vi "Add Server Information Refnums.vi"(8 "error in (no error)":errorcluster, 9 "Server Information Controls":refnum<vi>[](array[refnum]), 10 "Server URL":refnum<k21>, 11 "Map In":variant) -> (0 "error out":errorcluster, 3 "Map Out":variant)   [LabVIEW 2024]
doc: "Adds the mapping relationship between the server information variable URL and the control refnum to the map."
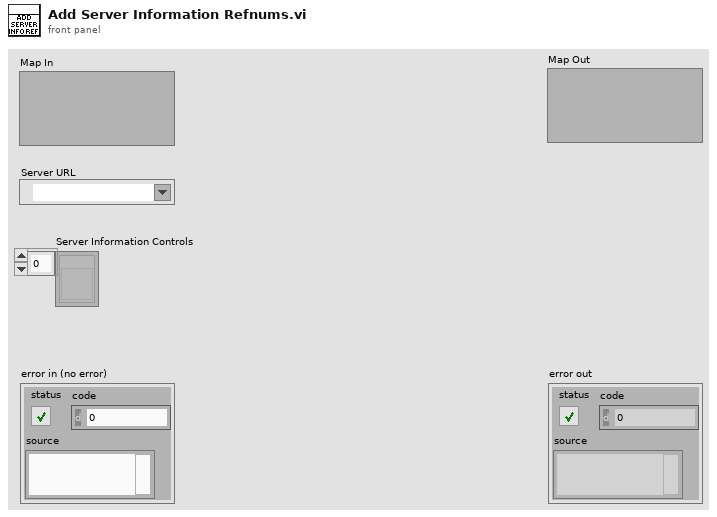
[diagram p1: front panel]
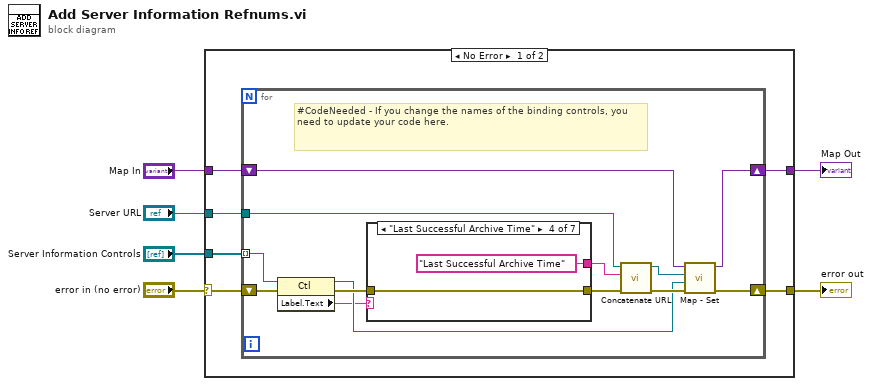
[diagram p0: block diagram]
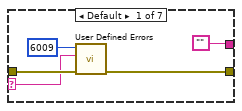
[diagram p2: hidden frame]
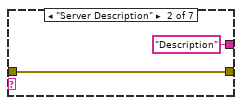
[diagram p3: hidden frame]
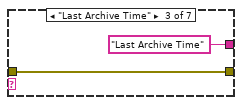
[diagram p4: hidden frame]
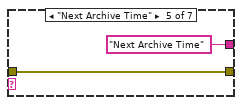
[diagram p5: hidden frame]
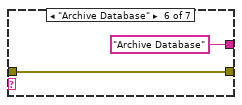
[diagram p6: hidden frame]
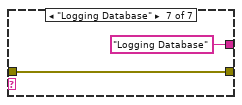
[diagram p7: hidden frame]
diagram:
  n1 = case shown="No Error" "error in (no error)" {
    selector: "error in (no error)" -> [w11 w44]
    tunnel: [w12 w44] -> w5
    tunnel: "Server URL" -> [w7 _]
    tunnel: "Map In" -> [w10 w43]
    tunnel: "Server Information Controls" -> [w9 _]
    tunnel: [w8 w43] -> w1
    frame No Error {
      n2 = for {
        tunnel: w9 -> [w17] mode=indexing
        shift-right: [w23] -> w12
        shift-left: w11 -> [w16]
        shift-right: [w24] -> w8
        shift-left: w10 -> [w25]
        tunnel: w7 -> [w19]
        # "#CodeNeeded - If you change the names of the binding controls, you need to update your code here."
        n3 = property class="Ctl"(reference=w17, error in=w16) -> (reference out=w14:refnum<vi>, error out=w15:errorcluster, "Label.Text"=w13:string)
        n4 = case shown="\"Last Successful Archive Time\"" w13 {
          selector: w13 -> [w27 _ _ _ _ _ _]
          tunnel: ["" "Description" ("string") "Last Archive Time" ("string") "Last Successful Archive Time" ("string") "Next Archive Time" ("string") "Archive Database" ("string") "Logging Database" ("string")] -> w18
          tunnel: [w29 w31 w33 w35 w37 w39 w41] -> w21
          tunnel: w15 -> [w28 w31 w33 w35 w37 w39 w41]
          frame Default {
            n5 = call "User Defined Errors.vi"("error in (no error)"=w28, "Parameter 1"=w27, "Error Code (0)"=6009 ("error code (0)")) -> ("error out"=w29:errorcluster)  [unwired: 8 in]
          }
          frame "Server Description" {
          }
          frame "Last Archive Time" {
          }
          frame "Last Successful Archive Time" {
          }
          frame "Next Archive Time" {
          }
          frame "Archive Database" {
          }
          frame "Logging Database" {
          }
        }
        n6 = call "Concatenate URL.vi"("error in (no error)"=w21, "Child Name"=w18, "Parent URL"=w19) -> ("error out"=w22:errorcluster, "Child URL"=w20:refnum<k21>)  [unwired: 7 in]
        n7 = call "Map - Set.vi"("error in (no error)"=w22, "Value"=w14, "Key"=w20, "Map In"=w25) -> ("error out"=w23:errorcluster, "Map Out"=w24:variant)  [unwired: 5 in, 1 out]
      }
    }
    frame Error {
    }
  }
  "error out" <- w5
  "Map Out" <- w1
